vi "autostage-coordinates-to-graph.vi"(1 "coordinates":dbl[][](array[numeric])) -> (0 "graph array":dbl[][](array[numeric]))   [LabVIEW 2017]
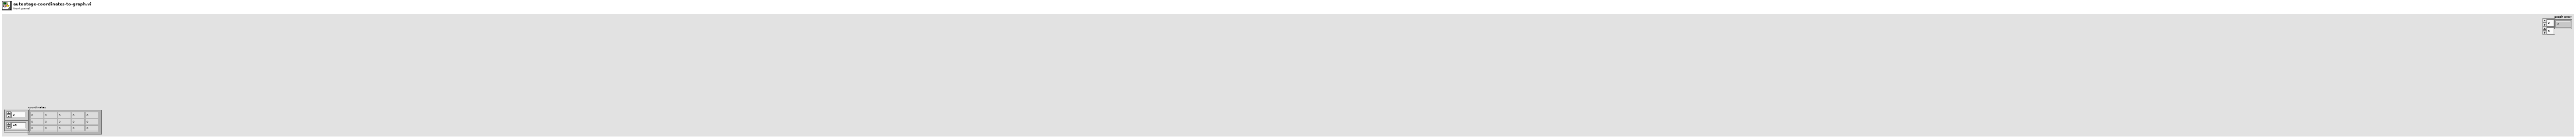
[diagram p1: front panel]
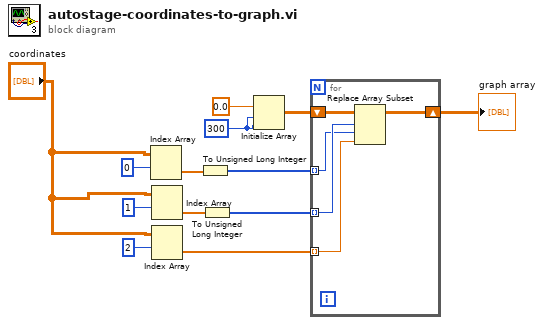
[diagram p0: block diagram]
diagram:
  w5 = 300 ("dimension size")
  n1 = Index Array(array="coordinates", index (row)=0) -> (element=w10:dbl[])  [unwired: 1 in]
  n2 = Index Array(array="coordinates", index (row)=1) -> (element=w12:dbl[])  [unwired: 1 in]
  n3 = Index Array(array="coordinates", index (row)=2) -> (element=w13:dbl[])  [unwired: 1 in]
  n4 = To Unsigned Long Integer(number=w10) -> (unsigned 32bit integer=w11:u32[])
  n5 = To Unsigned Long Integer(number=w12) -> (unsigned 32bit integer=w2:u32[])
  n6 = Initialize Array(0.0 ("element"), w5, w5) -> (w6:dbl[][])
  n7 = for {
    shift-right: [w17] -> w1
    shift-left: w6 -> [w18]
    tunnel: w11 -> [w14] mode=indexing
    tunnel: w2 -> [w15] mode=indexing
    tunnel: w13 -> [w16] mode=indexing
    n8 = Replace Array Subset(array=w18, new element=w16, index (row)=w15, index (col)=w14) -> (w17:dbl[][])
  }
  "graph array" <- w1
